vi "initialize.vi"(0 "HGF_SVVisitor_register":refnum<class "HGF_SVMonitorVisitor_register.lvclass">, 3 "initializationData":variant, 5 "error in (no error)":errorcluster, 7 "binaryString":string, 8 "I8 Array":i8[](array[numeric]), 9 "prependSize? (T)":bool, 11 "byteOrder (0:big-endian, network order)":T1(ring)) -> (14 "dup HGF_SVVisitor_register":refnum<class "HGF_SVMonitorVisitor_register.lvclass">, 17 "found?":bool, 19 "error out":errorcluster)   [LabVIEW 2012, in "HGF_SV.lvlib" / "HGF_SVMonitorVisitor_register.lvclass"]
doc: "This is a dynamic dispatch VI to be implemented by child classes to initialize their attributes.\n\n<B>Recommendation:</B> Use Variant for initialization data."
uses:
  HGF_SVMonitorVisitor_register.lvclass
  HGF_BaseClasses/HGF_NetworkVisitor/HGF_NetworkVisitor.lvclass
  HGF_BaseClasses/HGF_TriggeredEvent/HGF_TriggeredEvent.lvclass
  HGF_SVMonitorVisitor/HGF_SVMonitorVisitor.lvclass
  HGF_SVMonitorVisitor_register.lvclass/HGF_SVMonitorVisitor_register.ctl
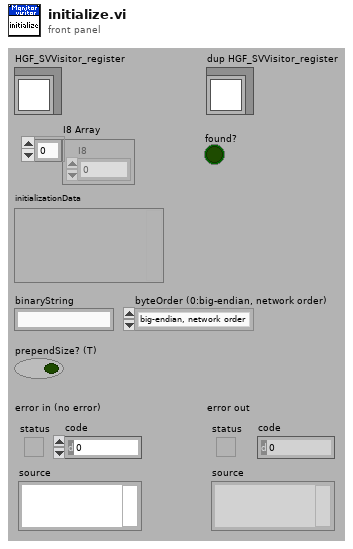
[diagram p1: front panel]
types:
  T1 = enum16{"big-endian, network order", "native, host order", "little-endian"}
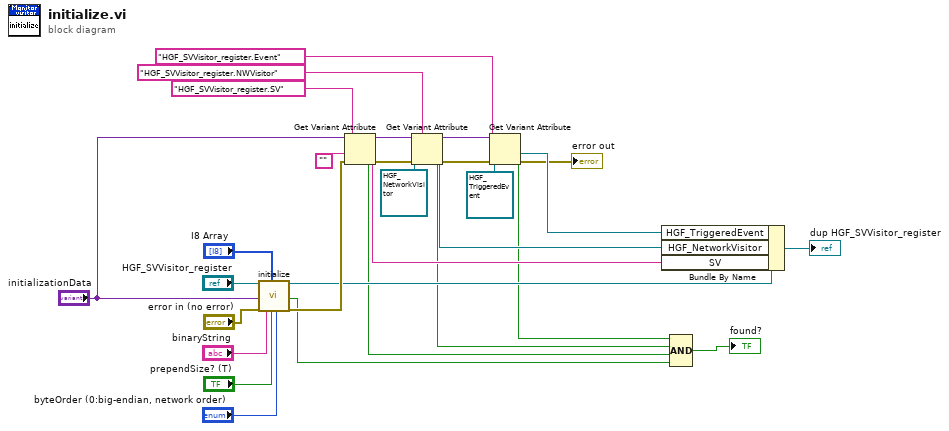
[diagram p0: block diagram]
diagram:
  n1 = call-parent "initialize.vi"("HGF_Visitor"="HGF_SVVisitor_register", "initializationData"="initializationData", "error in (no error)"="error in (no error)", "binaryString"="binaryString", "I8 Array"="I8 Array", "prependSize? (T)"="prependSize? (T)", "byteOrder (0:big-endian, network order)"="byteOrder (0:big-endian, network order)") -> ("dup HGF_Visitor"=w12:refnum<class "HGF_SVMonitorVisitor_register.lvclass">, "found?"=w7:bool, "error out"=w13:errorcluster)  [unwired: 10 in]
  n2 = Get Variant Attribute(Variant="initializationData", name="HGF_SVVisitor_register.SV", default value (empty Variant)="", error in=w13) -> (duplicate Variant=w17:variant, found=w5:bool, value=w10:string, error out=w23:errorcluster)
  n3 = Get Variant Attribute(Variant=w17, name="HGF_SVVisitor_register.NWVisitor", default value (empty Variant)=refnum<class "HGF_NetworkVisitor.lvclass"> refnum ("HGF_NetworkVisitor"), error in=w23) -> (duplicate Variant=w18:variant, found=w4:bool, value=w9:refnum<class "HGF_NetworkVisitor.lvclass">, error out=w22:errorcluster)
  n4 = Get Variant Attribute(Variant=w18, name="HGF_SVVisitor_register.Event", default value (empty Variant)=refnum<class "HGF_TriggeredEvent.lvclass"> refnum ("HGF_BaseClasses.lvlib:HGF_TriggeredEvent.lvclass"), error in=w22) -> (found=w3:bool, value=w6:refnum<class "HGF_TriggeredEvent.lvclass">, error out=→"error out":errorcluster)  [unwired: 1 out]
  n5 = Bundle By Name(cluster=w12, "HGF_TriggeredEvent"=w6, "HGF_NetworkVisitor"=w9, "SV"=w10) -> (→"dup HGF_SVVisitor_register":refnum<class "HGF_SVMonitorVisitor_register.lvclass">)
  n6 = Compound Arithmetic op=AND(w3, w4, w5, w7) -> (→"found?":bool)
